vi "BarLIV_Ex_DataOut_autoReport1.vi"(2 "error in (no error)":errorcluster, 3 "Bar_LIV_AutoRep":path=path "D:/LabVIEW_prog/Trumpf_Database_Connect/DM17_TestFiles_AutoReport/30082943autoreport_Pre_05-31-2019_10-11-46.xlsx") -> (0 "error out":errorcluster={"status"=TRUE, "code"=7, "source"="NI_Excel.lvclass:new report subVI.vi -> NI_report.lvclass:New Report.vi -> BarLIV_Ex_DataOut_autoReport.vi\r\n"}, 1 "BarLIV AutoRep Output":T1={"Date"="12/30/1899", "LIV Data"=[], "Polarization"=0.0, "Bar SN"="", "Bar WO"="", "Wafer ID"=""})   [LabVIEW 2017]
uses:
  <vilib>/addons/_office/excel.llb/Excel Get Data (str).vi
  <vilib>/addons/_office/excel.llb/Excel Get Data ([dbl]).vi
  <vilib>/addons/_office/excel.llb/Excel Get Data (dbl).vi
  <vilib>/Utility/NIReport.llb/NI_report.lvclass
  <vilib>/addons/_office/NI_ReportGenerationToolkit.lvlib
  <vilib>/Utility/NIReport.llb/Excel/NI_Excel.lvclass
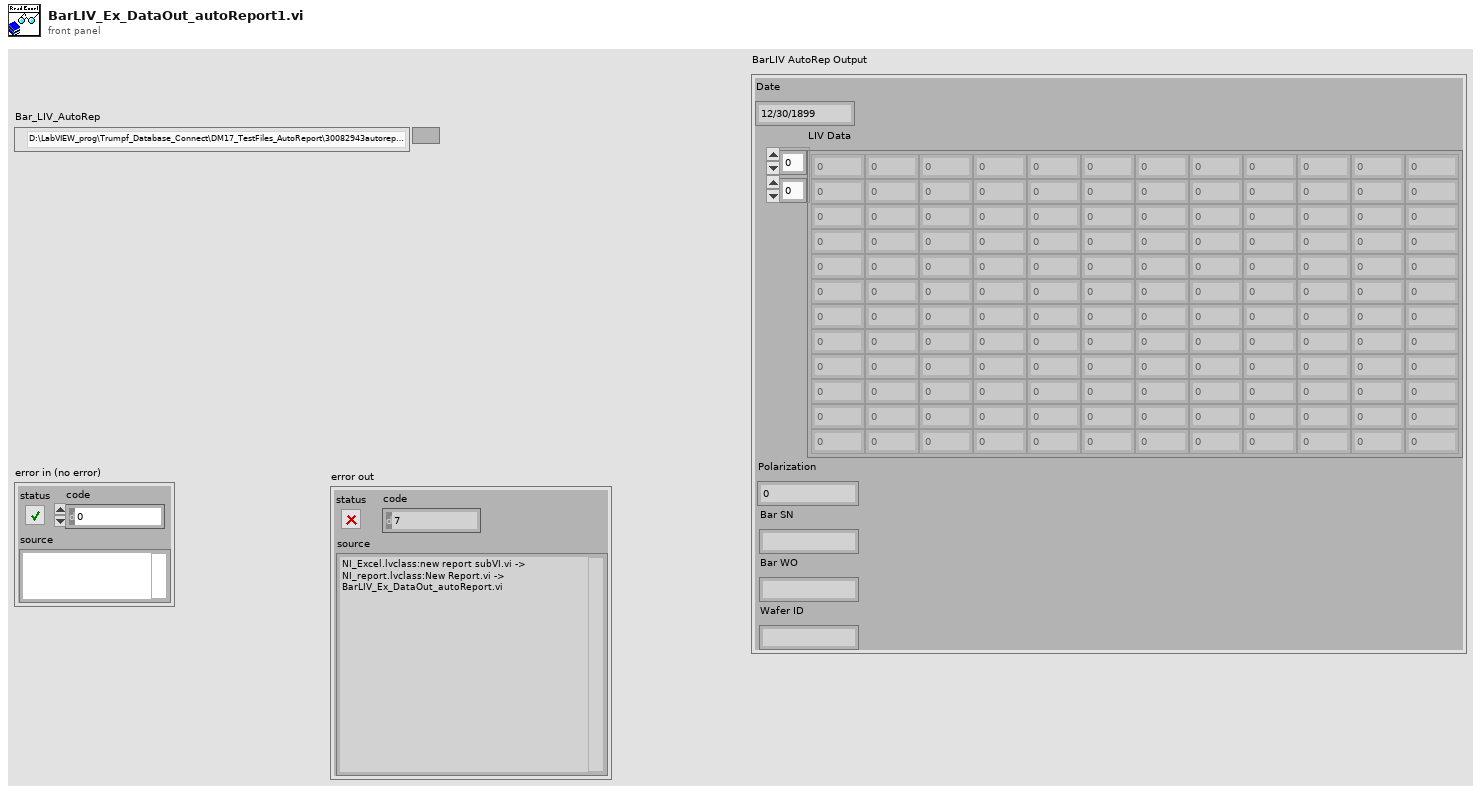
[diagram p1: front panel]
types:
  T1 = cluster{"Date":string, "LIV Data":dbl[][], "Polarization":dbl, "Bar SN":string, "Bar WO":string, "Wafer ID":string}
  T2 = enum16{"Standard Report", "HTML", "Word", "Excel"}
  T3 = cluster{"date/time string":string, "data":dbl[][], dbl, "data":string, "data":string, "data":string}
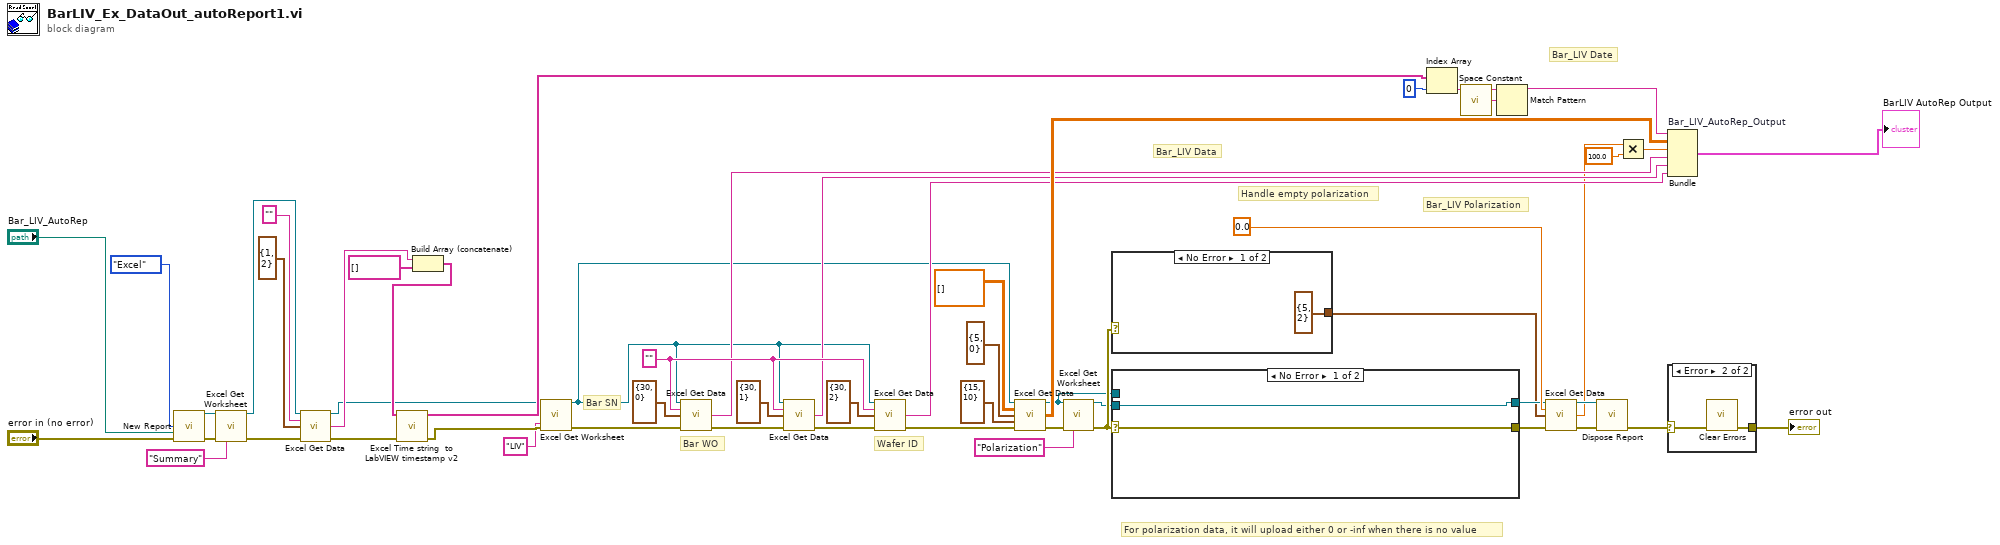
[diagram p0: block diagram]
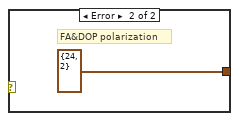
[diagram p3: hidden frame]
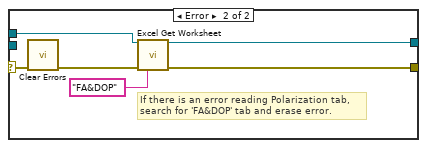
[diagram p4: hidden frame]
diagram:
  w22 = ""
  # "For polarization data, it will upload either 0 or -inf when there is no value"
  # "Wafer ID"
  # "Bar WO"
  # "Bar SN"
  # "Handle empty polarization"
  # "Bar_LIV Polarization"
  # "Bar_LIV Date"
  # "Bar_LIV Data"
  n1 = call <vilib>:"New Report.vi"("report type"=T2."Excel", "template (empty)"="Bar_LIV_AutoRep", "error in (no error)"="error in (no error)") -> ("report out"=w53:refnum<class "NI_report.lvclass">, "error out"=w52:errorcluster)  [unwired: 11 in]
  n2 = call <vilib>:"Excel Get Worksheet.vi"("report in"=w53, "error in (no error)"=w52, "name (\"\")"="Summary" ("name (\"\")")) -> ("report out"=w50:refnum<class "NI_report.lvclass">, "error out"=w48:errorcluster)  [unwired: 1 in, 10 out]
  n3 = call-poly <vilib>:"Excel Get Data.vi"("report in"=w50, "data type"="", "start (0, 0)"=cluster{"start row":i32, "start column":i32} {"start row"=1, "start column"=2}, "error in (no error)"=w48) -> ("report out"=w40:refnum<class "NI_report.lvclass">, "data"=w45:string, "error out"=w43:errorcluster)  [unwired: 9 in]
  n4 = Build Array (concatenate)(w45, string[] []) -> (w44:string[])
  n5 = call "Excel Time string  to LabVIEW timestamp v2.vi"("Error In"=w43, "XLDateIn"=w44) -> ("Error Out"=w39:errorcluster, "DateOut"=w41:string[])  [unwired: 7 in, 1 out]
  n6 = call <vilib>:"Excel Get Worksheet.vi"("report in"=w40, "error in (no error)"=w39, "name (\"\")"="LIV" ("name (\"\")")) -> ("report out"=w6:refnum<class "NI_report.lvclass">, "error out"=w18:errorcluster)  [unwired: 1 in, 10 out]
  n7 = call-poly <vilib>:"Excel Get Data.vi"("report in"=w6, "data type"=w22, "start (0, 0)"=cluster{"start row":i32, "start column":i32} {"start row"=30, "start column"=0}, "error in (no error)"=w18) -> ("data"=w14:string, "error out"=w17:errorcluster)  [unwired: 9 in, 1 out]
  n8 = call-poly <vilib>:"Excel Get Data.vi"("report in"=w6, "data type"=w22, "start (0, 0)"=cluster{"start row":i32, "start column":i32} {"start row"=30, "start column"=1}, "error in (no error)"=w17) -> ("data"=w13:string, "error out"=w16:errorcluster)  [unwired: 9 in, 1 out]
  n9 = call-poly <vilib>:"Excel Get Data.vi"("report in"=w6, "data type"=w22, "start (0, 0)"=cluster{"start row":i32, "start column":i32} {"start row"=30, "start column"=2}, "error in (no error)"=w16) -> ("data"=w12:string, "error out"=w15:errorcluster)  [unwired: 9 in, 1 out]
  n10 = call-poly <vilib>:"Excel Get Data.vi"("report in"=w6, "data type"=dbl[][] [], "start (-1, -1)"=cluster{"row":i32, "column":i32} {"row"=5, "column"=0}, "end (-1, -1)"=cluster{"row":i32, "column":i32} {"row"=15, "column"=10}, "error in (no error)"=w15) -> ("report out"=w5:refnum<class "NI_report.lvclass">, "data"=w34:dbl[][], "error out"=w33:errorcluster)  [unwired: 8 in]
  n11 = call <vilib>:"Excel Get Worksheet.vi"("report in"=w5, "error in (no error)"=w33, "name (\"\")"="Polarization" ("name (\"\")")) -> ("report out"=w4:refnum<class "NI_report.lvclass">, "error out"=w8:errorcluster)  [unwired: 1 in, 10 out]
  n12 = case shown="No Error" w8 {
    tunnel: [cluster{"row":i32, "column":i32} {"row"=5, "column"=2} ("start (-1, -1)") cluster{"row":i32, "column":i32} {"row"=24, "column"=2} ("start (-1, -1)")] -> w7
    frame No Error {
    }
    frame Error {
      # "FA&DOP polarization"
    }
  }
  n13 = case shown="No Error" w8 {
    selector: w8 -> [w59 w65]
    tunnel: [w59 w61] -> w10
    tunnel: w5 -> [_ w60]
    tunnel: [w58 w62] -> w9
    tunnel: w4 -> [w58 _]
    frame No Error {
    }
    frame Error {
      # "If there is an error reading Polarization tab, \nsearch for 'FA&DOP' tab and erase error."
      n14 = call <vilib>:"Clear Errors.vi"("error in (no error)"=w65) -> ("error out"=w64:errorcluster)  [unwired: 5 in, 1 out]
      n15 = call <vilib>:"Excel Get Worksheet.vi"("report in"=w60, "error in (no error)"=w64, "name (\"\")"="FA&DOP" ("name (\"\")")) -> ("report out"=w62:refnum<class "NI_report.lvclass">, "error out"=w61:errorcluster)  [unwired: 1 in, 10 out]
    }
  }
  n16 = Index Array(array=w41, index=0) -> (element=w26:string)
  n17 = call <vilib>:"Space Constant.vi"() -> ("String"=w25:string)
  n18 = Match Pattern(string=w26, regular expression=w25) -> (before substring=w24:string)  [unwired: 1 in, 3 out]
  n19 = call-poly <vilib>:"Excel Get Data.vi"("report in"=w9, "data type"=0.0, "start (0, 0)"=w7, "error in (no error)"=w10) -> ("report out"=w30:refnum<class "NI_report.lvclass">, "data"=w1:dbl, "error out"=w23:errorcluster)  [unwired: 9 in]
  n20 = call-dynamic "Dispose Report.vi"("report in"=w30, "error in (no error)"=w23) -> ("error out"=w3:errorcluster)  [unwired: 13 in]
  n21 = Multiply(x=w1, y=100.0) -> (x*y=w27:dbl)
  n22 = Bundle "Bar_LIV_AutoRep_Output"("date/time string"=w24, "data"=w34, w27, "data"=w14, "data"=w13, "data"=w12) -> (→"BarLIV AutoRep Output":T3)  [unwired: 1 in]
  n23 = case shown="Error" w3 {
    selector: w3 -> [w66 w68]
    tunnel: [w66 w67] -> w2
    frame No Error {
    }
    frame Error {
      n24 = call <vilib>:"Clear Errors.vi"("error in (no error)"=w68) -> ("error out"=w67:errorcluster)  [unwired: 5 in, 1 out]
    }
  }
  "error out" <- w2
